vi "模式切换.vi"() -> ()   [LabVIEW 2020]
uses:
  Global_Variable/Global.vi
panel:
  in  "单选按钮":enum32{"单机", "追溯"}(radio)
  # "模式切换"
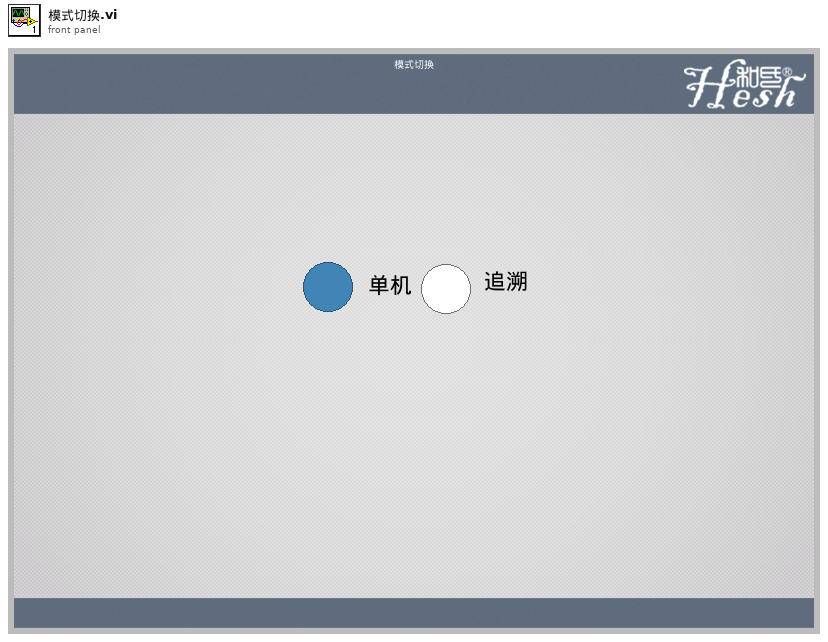
[diagram p1: front panel]
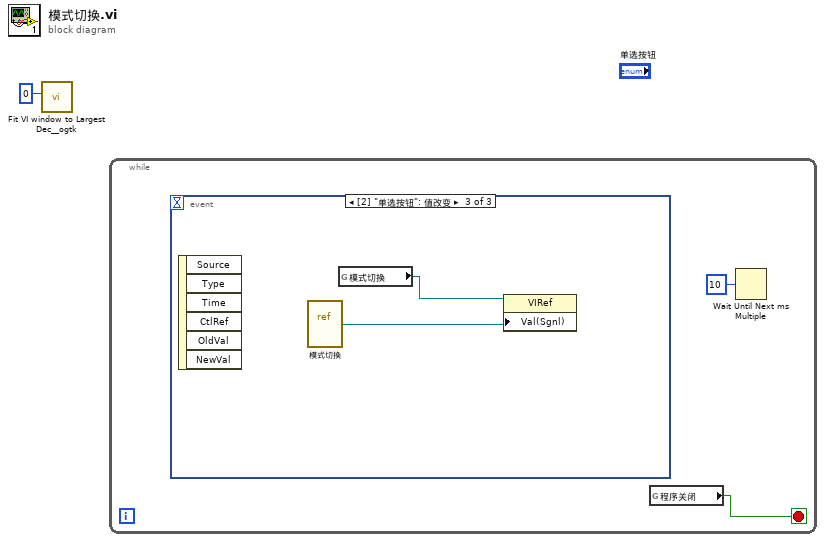
[diagram p0: block diagram]
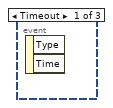
[diagram p2: hidden frame]
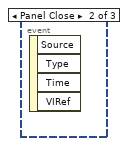
[diagram p3: hidden frame]
diagram:
  n1 = call <userlib>:"Fit VI window to Largest Dec__ogtk.vi"("border spacing (2 px)"=0) -> ()  [unwired: 5 in, 2 out]
  n2 = while {
    stop <- w3 stop-if-true
    n3 = event shown="[2] \"单选按钮\": 值改变" {
      selector: _ -> [_ _ _]
      dyn-events: _ -> [_ _ _]
      timeout: _ -> [_ _ _]
      event Timeout {
        n4 = event-data() -> ()  [unwired: 1 in, 2 out]
      }
      event Panel Close {
        n5 = event-data() -> ()  [unwired: 1 in, 4 out]
      }
      event "单选按钮": Value Change {
        n6 = event-data() -> ()  [unwired: 1 in, 6 out]
        n7 = vi-ref "模式切换.vi"() -> (w4:refnum<vi>)
        n8 = global read "Global.vi" "模式切换"() -> (w5:refnum<vi>)
        n9 = property class="VIRef"(reference=w5, "Val(Sgnl)"=w4) -> ()  [unwired: 1 in, 2 out]
      }
    }
    n10 = global read "Global.vi" "程序关闭"() -> (w3:bool)
    n11 = Wait Until Next ms Multiple(millisecond multiple=u32 10 ("毫秒倍数")) -> ()  [unwired: 1 out]
  }
